vi "型号到特定类(源)转换.vi"(8 "error in (no error)":errorcluster caption="错误输入（无错误）", 11 "型号":string) -> (0 "错误输出":errorcluster, 3 "MC":refnum<class "多功能校准源接口.lvclass">)   [LabVIEW 2020]
uses:
  <vilib>/Utility/LVLibp/NI_PackedLibraryUtility.lvlib
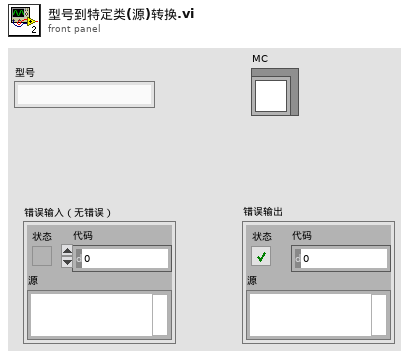
[diagram p1: front panel]
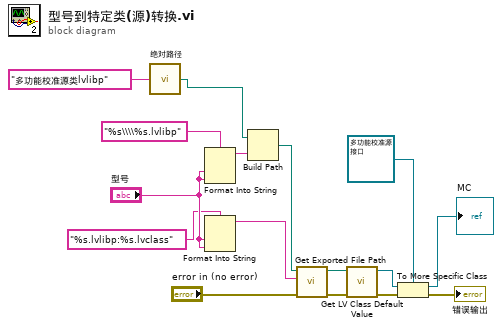
[diagram p0: block diagram]
diagram:
  n1 = call "绝对路径.vi"("相对路径"="多功能校准源类lvlibp" ("名称或相对路径")) -> ("绝对路径"=w3:path)
  n2 = Format Into String(format string="%s\\\\%s.lvlibp" ("名称或相对路径"), "型号", "型号") -> (resulting string=w10:string)  [unwired: 2 in, 1 out]
  n3 = Format Into String(format string="%s.lvlibp:%s.lvclass" ("名称或相对路径"), "型号", "型号") -> (resulting string=w12:string)  [unwired: 2 in, 1 out]
  n4 = Build Path(base path=w3, name or relative path=w10) -> (appended path=w11:path)
  n5 = call <vilib>:"Get Exported File Path.vi"("error in (no error)"="error in (no error)", "qualified name"=w12, "packed library path"=w11) -> ("error out"=w14:errorcluster, "path"=w13:path)  [unwired: 7 in]
  n6 = call <vilib>:"Get LV Class Default Value.vi"("error in (no error)"=w14, "class path"=w13) -> ("error out"=w16:errorcluster, "object"=w15:refnum<class>)  [unwired: 8 in]
  n7 = To More Specific Class(target class=refnum<class "多功能校准源接口.lvclass"> refnum ("多功能校准源接口.lvlibp:多功能校准源接口.lvclass"), reference=w15, error in=w16) -> (specific class reference=→"MC":refnum<class "多功能校准源接口.lvclass">, error out=→"错误输出":errorcluster)
